vi "PhotonPipelineResult_SetTimeStampSecs.vi"(9 "TimeStampSec":dbl, 11 "PhotonPipelineResult":T1 {"Targets"."AltCameraToTarget"."TRANSLATION3D"."Z" format="%14.3f"; "Targets"."AltCameraToTarget"."TRANSLATION3D"."Y" format="%14.3f"; "Targets"."AltCameraToTarget"."TRANSLATION3D"."X" format="%14.3f"; "Targets"."BestCameraToTarget"."TRANSLATION3D"."Z" format="%14.3f"; "Targets"."BestCameraToTarget"."TRANSLATION3D"."Y" format="%14.3f"; "Targets"."BestCameraToTarget"."TRANSLATION3D"."X" format="%14.3f"}) -> (3 "Out PhotonPipelineResult":T1 {"Targets"."AltCameraToTarget"."TRANSLATION3D"."Z" format="%14.3f"; "Targets"."AltCameraToTarget"."TRANSLATION3D"."Y" format="%14.3f"; "Targets"."AltCameraToTarget"."TRANSLATION3D"."X" format="%14.3f"; "Targets"."BestCameraToTarget"."TRANSLATION3D"."Z" format="%14.3f"; "Targets"."BestCameraToTarget"."TRANSLATION3D"."Y" format="%14.3f"; "Targets"."BestCameraToTarget"."TRANSLATION3D"."X" format="%14.3f"})   [LabVIEW 2019, in "PhotonVisionLib.lvlib"]
doc: "Returns pipeline packet time stamp\n\nInputs:\n - PipelineResult -- Parsed PipelineResult cluster.\n - TimeStampSec -- Time stamp of packet (FPGA elapsed time) seconds\n\nOutputs:\n - Out PipelineResult -- Updated PipelineResult cluster."
uses:
  TypeDef/PhotonPipelineResultType.ctl
  TypeDef/PhotonTrackedTargetType.ctl
  TypeDef/TargetCornerType.ctl
  <vilib>/Rock Robotics/WPI/ThirdParty/JAS_Junk/TrajLib/TypeDef/TRANSFORM3D.ctl
  <vilib>/Rock Robotics/WPI/ThirdParty/JAS_Junk/TrajLib/TypeDef/TRANSLATION3D.ctl
  <vilib>/Rock Robotics/WPI/ThirdParty/JAS_Junk/TrajLib/TypeDef/ROTATION3D.ctl
  <vilib>/Rock Robotics/WPI/ThirdParty/JAS_Junk/TrajLib/TypeDef/QUATERNION.ctl
  PhotonVisionLib.lvlib
  <vilib>/Rock Robotics/WPI/ThirdParty/JAS_Junk/TrajLib/Trajectory_Library.lvlib
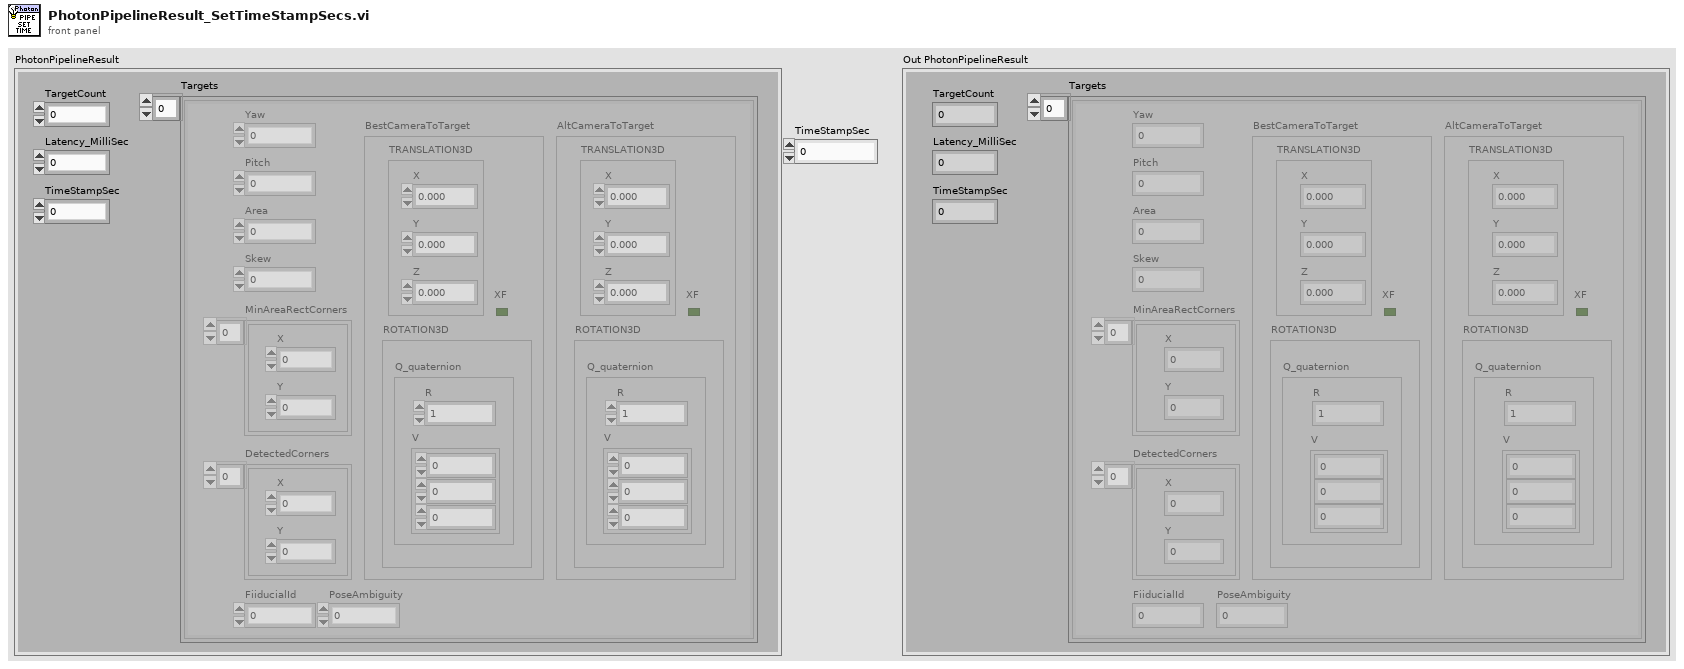
[diagram p1: front panel]
types:
  T1 = typedef "PhotonVisionLib.lvlib/PhotonPipelineResultType.ctl" = cluster{"TargetCount":i32, "Latency_MilliSec":dbl, "Targets":T2[], "TimeStampSec":dbl}
  T2 = typedef "PhotonVisionLib.lvlib/PhotonTrackedTargetType.ctl" = cluster{"Yaw":dbl, "Pitch":dbl, "Area":dbl, "Skew":dbl, "MinAreaRectCorners":T3[], "BestCameraToTarget":T4, "FiiducialId":i32, "AltCameraToTarget":T4, "PoseAmbiguity":dbl, "DetectedCorners":T3[]}
  T3 = typedef "PhotonVisionLib.lvlib/TargetCornerType.ctl" = cluster{"X":dbl, "Y":dbl}
  T4 = typedef "Trajectory_Library.lvlib/TRANSFORM3D.ctl" = cluster{"TRANSLATION3D":T5, "ROTATION3D":T6, "XF":bool}
  T5 = typedef "Trajectory_Library.lvlib/TRANSLATION3D.ctl" = cluster{"X":dbl, "Y":dbl, "Z":dbl}
  T6 = typedef "Trajectory_Library.lvlib/ROTATION3D.ctl" = cluster{"Q_quaternion":T7}
  T7 = typedef "Trajectory_Library.lvlib/QUATERNION.ctl" = cluster{"R":dbl, "V":dbl[]}
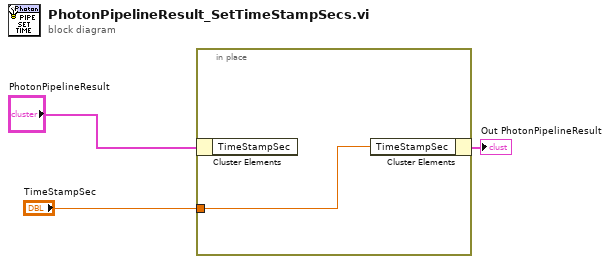
[diagram p0: block diagram]
diagram:
  n1 = in-place {
    in-place-border: "TimeStampSec" -> [w4]
    n2 = in-place-cluster #1("PhotonPipelineResult") -> ()  [unwired: 1 out]
    n3 = in-place-cluster #1("TimeStampSec"=w4) -> (→"Out PhotonPipelineResult":T1)
  }
